vi "getMicSensitivity.vi"(10 "Ref.Frequenz":dbl=100.0, 11 "fundamental amplitude":T1) -> (3 "Sensitivity/V":dbl)   [LabVIEW 2012]
doc: "Holt den Spannungswert einer bestimmten Frequenz aus dem Container.\nDie exakte Frequenz muss Teil der Frequenzliste sein."
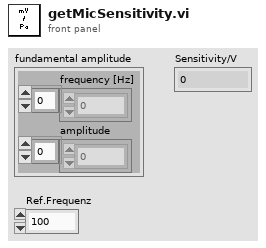
[diagram p1: front panel]
types:
  T1 = cluster{"frequency [Hz]":dbl[], "amplitude":dbl[]}
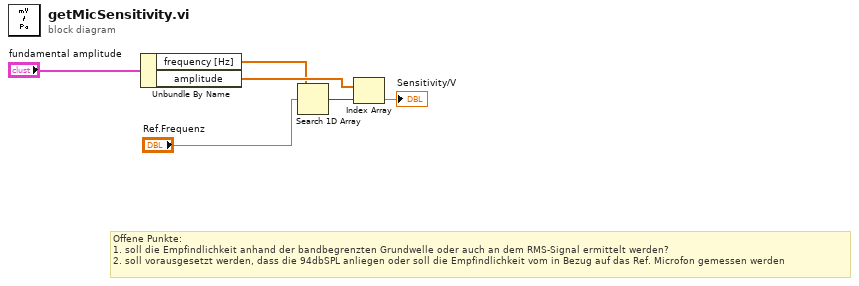
[diagram p0: block diagram]
diagram:
  # "Offene Punkte:\n1. soll die Empfindlichkeit anhand der bandbegrenzten Grundwelle oder auch an dem RMS-Signal ermittelt werden?\n2. soll vorausgesetzt werden, dass die 94dbSPL anliegen oder soll die Empfindlichkeit vom in Bezug auf das Ref. Microfon gemessen werden"
  n1 = Unbundle By Name("fundamental amplitude") -> ("frequency [Hz]"=w2:dbl[], "amplitude"=w5:dbl[])
  n2 = Search 1D Array(1D array=w2, element="Ref.Frequenz") -> (index of element=w4:i32)  [unwired: 1 in]
  n3 = Index Array(array=w5, index=w4) -> (element=→"Sensitivity/V":dbl)
